vi "InitDevices.vi"(9 "Stanford ID":refnum<visa-resource-name>, 11 "Keithley ID":refnum<visa-resource-name>) -> (0 "Stanford Err":errorcluster, 1 "Stanford ID":refnum<visa-resource-name>, 2 "Keithley Err":errorcluster, 3 "Keithley ID":refnum<visa-resource-name>)   [LabVIEW 2013]
uses:
  StanfordVoltage.vi
  IntegrationTime-global.vi
  <instrlib>/Keithley 24XX/Keithley 24XX.lvlib
  <instrlib>/Stanford Research 830/Stanford Research 830.lvlib
panel:
  out "Time Constant (8: 100ms) 2":u16(ring)=8 items=["10 us", "30 us", "100 us", "300 us", "1 ms", "3 ms", "10 ms", "30 ms", "100 ms", "300 ms", "1 s", "3 s", "10 s", "30 s", "100 s", "300 s", "1 ks", "3 ks", "10 ks", "30 ks"]
  in  "Low Pass Filter Slope (1: 12dB/oct)":u16(ring)=1 items=["6 dB/oct", "12 dB/oct", "18 db/oct", "24 dB/oct"]
  in  "Time Constant (8: 100ms)":u16(ring)=8 items=["10 us", "30 us", "100 us", "300 us", "1 ms", "3 ms", "10 ms", "30 ms", "100 ms", "300 ms", "1 s", "3 s", "10 s", "30 s", "100 s", "300 s", "1 ks", "3 ks", "10 ks", "30 ks"]
  in  "Internal Reference Frequency (1000 Hz)":dbl=1000.0
  in  "Sine Output Amplitude (1 V)":dbl=1.0
  in  "Sensitivity (26: 1 V/uA)":i16(ring)=-1 items=["Auto Gain"=-1, "2 nV/fA"=0, "5 nV/fA"=1, "10 nV/fA"=2, "20 nV/fA"=3, "50 nV/fA"=4, "100 nV/fA"=5, "200 nV/fA"=6, "500 nV/fA"=7, "1 uV/pA"=8, "2 uV/pA"=9, "5 uV/pA"=10, "10 uV/pA"=11, "20 uV/pA"=12, "50 uV/pA"=13, "100 uV/pA"=14, "200 uV/pA"=15, "500 uV/pA"=16, "1 mV/nA"=17, "2 mV/nA"=18, "5 mV/nA"=19, "10 mV/nA"=20, "20 mV/nA"=21, "50 mV/nA"=22, "100 mV/nA"=23, "200 mV/nA"=24, "500 mV/mA"=25, "1 V/uA"=26]
  in  "Dynamic Reserve (2: Low Noise)":i16(ring)=2 items=["High Reserve"=0, "Normal"=1, "Low Noise"=2, "Auto Reserve"=-1]
  in  "Reference Source (1: Internal)":u16(ring)=1 items=["External", "Internal"]
  in  "Input Coupling (0: AC)":u16(ring) items=["AC", "DC"]
  in  "Input Connection (0: Single-Ended Voltage)":u16(ring) items=["Single-Ended Voltage", "Differential Voltage", "1 MOhm Current Gain", "100 MOhm Current Gain"]
  # "LOCK IN"
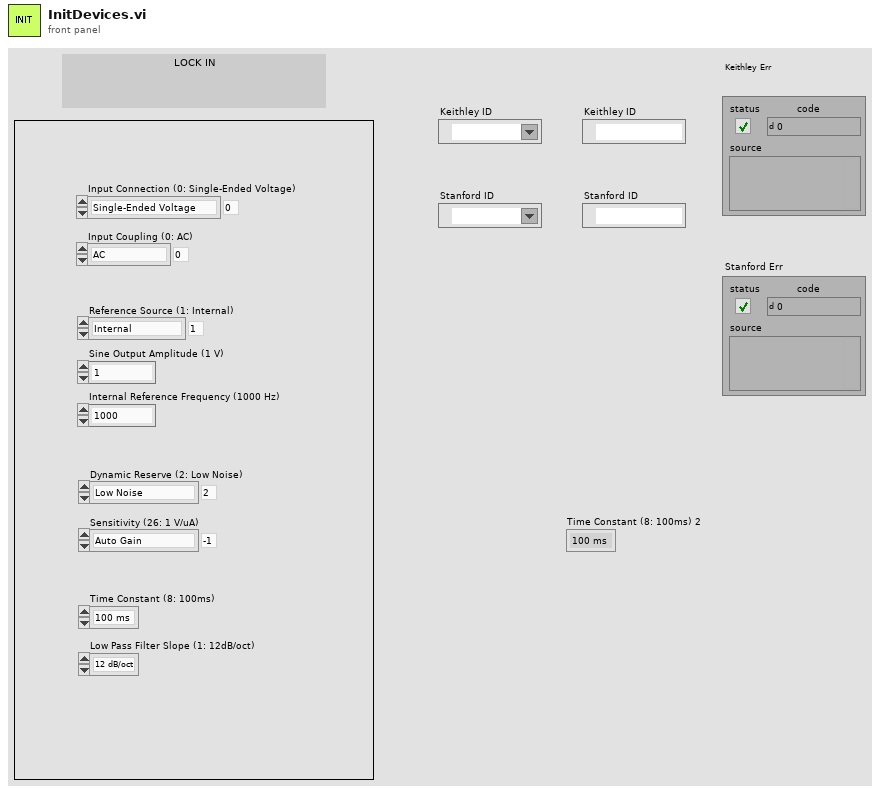
[diagram p1: front panel]
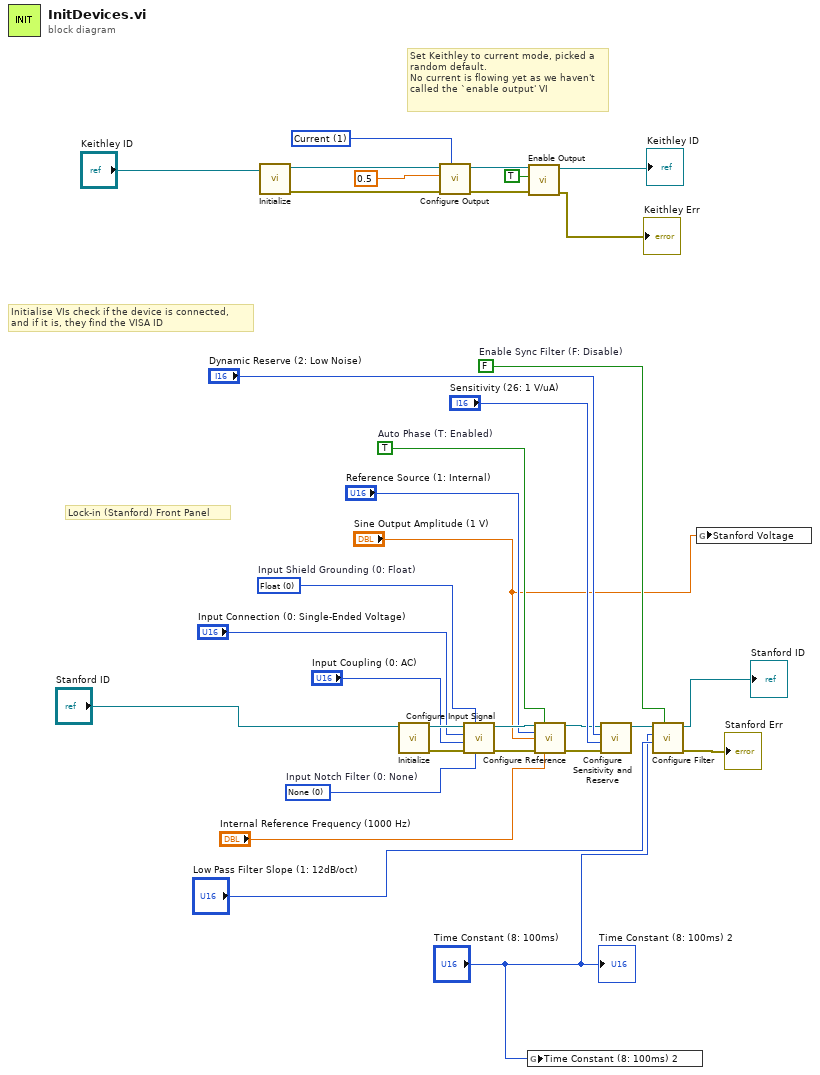
[diagram p0: block diagram]
diagram:
  w11 = FALSE  # Enable Sync Filter (F: Disable)
  w20 = TRUE  # Auto Phase (T: Enabled)
  w21 = u16 0 items=["None", "Line Notch", "2x Line Notch", "Both Notch Filters"]  # Input Notch Filter (0: None)
  w22 = u16 0 items=["Float", "Ground"]  # Input Shield Grounding (0: Float)
  w32 = u16 1 items=["Voltage", "Current"] ("Source Mode  (0: Voltage)")
  # "Lock-in (Stanford) Front Panel"
  # "Set Keithley to current mode, picked a random default.\nNo current is flowing yet as we haven't called the `enable output' VI"
  # "Initialise VIs check if the device is connected, \nand if it is, they find the VISA ID"
  n1 = call <instrlib>:"Initialize.vi"("VISA resource name"="Keithley ID") -> ("error out"=w30:errorcluster, "VISA resource name out"=w33:refnum<visa-resource-name>)  [unwired: 9 in]
  n2 = call <instrlib>:"Initialize.vi"("VISA resource name"="Stanford ID") -> ("error out"=w28:errorcluster, "VISA resource name out"=w27:refnum<visa-resource-name>)  [unwired: 9 in]
  n3 = call <instrlib>:"Configure Output.vi"("Source Mode  (0: Voltage)"=w32, "error in (no error)"=w30, "Output Level (0)"=0.5, "VISA resource name"=w33) -> ("error out"=w6:errorcluster, "VISA resource name out"=w7:refnum<visa-resource-name>)  [unwired: 6 in]
  n4 = call <instrlib>:"Configure Input Signal.vi"("Input Notch Filter (0: None)"=w21, "Input Shield Grounding (0: Float)"=w22, "error in (no error)"=w28, "Input Coupling (0: AC)"="Input Coupling (0: AC)", "Input Connection (0: Single-Ended Voltage)"="Input Connection (0: Single-Ended Voltage)", "VISA resource name"=w27) -> ("error out"=w25:errorcluster, "VISA resource name out"=w26:refnum<visa-resource-name>)  [unwired: 4 in]
  n5 = global write "IntegrationTime-global.vi" "Time Constant (8: 100ms) 2"("Time Constant (8: 100ms)") -> ()
  n6 = call <instrlib>:"Enable Output.vi"("error in (no error)"=w6, "Enable Output (T: Enable)"=TRUE, "VISA resource name"=w7) -> ("error out"=→"Keithley Err":errorcluster, "VISA resource name out"=→"Keithley ID":refnum<visa-resource-name>)  [unwired: 7 in]
  n7 = call <instrlib>:"Configure Reference.vi"("VISA resource name"=w26, "Auto Phase (T: Enabled)"=w20, "Reference Source (1: Internal)"="Reference Source (1: Internal)", "Sine Output Amplitude (1 V)"="Sine Output Amplitude (1 V)", "error in (no error)"=w25, "Internal Reference Frequency (1000 Hz)"="Internal Reference Frequency (1000 Hz)") -> ("VISA resource name out"=w17:refnum<visa-resource-name>, "error out"=w16:errorcluster)  [unwired: 8 in]
  n8 = call <instrlib>:"Configure Sensitivity and Reserve.vi"("error in (no error)"=w16, "Sensitivity (-1: Auto gain)"="Sensitivity (26: 1 V/uA)", "Dynamic Reserve (-1: Auto Reserve)"="Dynamic Reserve (2: Low Noise)", "VISA resource name"=w17) -> ("VISA resource name out"=w13:refnum<visa-resource-name>)  [unwired: 6 in, 1 out]
  n9 = call <instrlib>:"Configure Filter.vi"("Enable Sync Filter (F: Disable)"=w11, "Low Pass Filter Slope (1: 12dB/oct)"="Low Pass Filter Slope (1: 12dB/oct)", "Time Constant (8: 100ms)"="Time Constant (8: 100ms)", "VISA resource name"=w13) -> ("error out"=→"Stanford Err":errorcluster, "VISA resource name out"=→"Stanford ID":refnum<visa-resource-name>)  [unwired: 6 in]
  n10 = global write "StanfordVoltage.vi" "Stanford Voltage"("Sine Output Amplitude (1 V)") -> ()
  "Time Constant (8: 100ms) 2" <- "Time Constant (8: 100ms)"
